vi "Day 8.1 - .vi"(11 "input":i32[][](array[numeric])) -> (3 "output":i16)   [LabVIEW 2021]
panel:
  out "Array":bool[][](array[boolean])
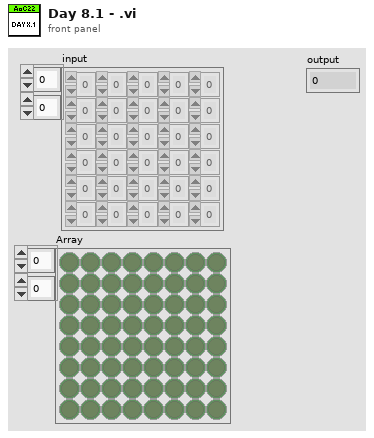
[diagram p1: front panel]
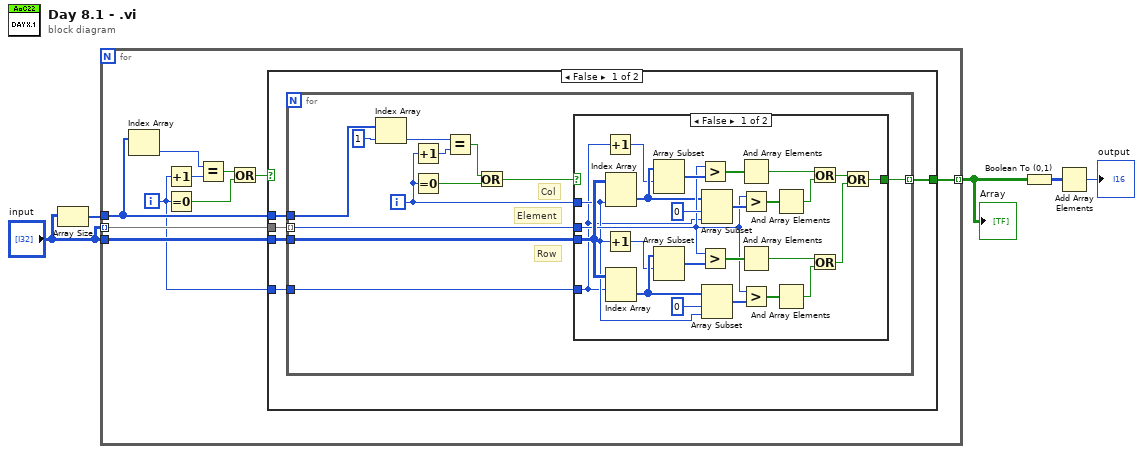
[diagram p0: block diagram]
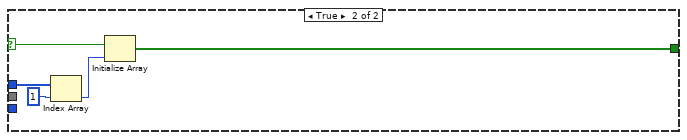
[diagram p3: hidden frame]
diagram:
  n1 = Array Size(array="input") -> (size(s)=w4:i32[])
  n2 = for {
    tunnel: "input" -> [w15] mode=indexing
    tunnel: "input" -> [w14]
    tunnel: w4 -> [w13]
    tunnel: [w7] -> w3 mode=indexing
    i -> [w6]
    n3 = Index Array(array=w13) -> (element=w12:i32)  [unwired: 1 in]
    n4 = Increment(x=w6) -> (x+1=w11:i32)
    n5 = Equal To 0?(x=w6) -> (x = 0?=w9:bool)
    n6 = Equal?(x=w12, y=w11) -> (x = y?=w10:bool)
    n7 = Or(x=w10, y=w9) -> (x .or. y?=w8:bool)
    n8 = case shown="False" w8 {
      selector: w8 -> [_ w63]
      tunnel: w15 -> [w20 _]
      tunnel: w14 -> [w19 _]
      tunnel: w13 -> [w18 w59]
      tunnel: [w17 w62] -> w7
      tunnel: w6 -> [w16 _]
      frame False {
        n9 = for {
          tunnel: w20 -> [w23] mode=indexing
          tunnel: w19 -> [w24]
          tunnel: w18 -> [w28]
          tunnel: [w25] -> w17 mode=indexing
          tunnel: w16 -> [w21]
          i -> [w22]
          # "Col"
          # "Row"
          # "Element"
          n10 = Index Array(array=w28, index=1) -> (element=w29:i32)
          n11 = Increment(x=w22) -> (x+1=w30:i32)
          n12 = Equal To 0?(x=w22) -> (x = 0?=w32:bool)
          n13 = Equal?(x=w29, y=w30) -> (x = y?=w31:bool)
          n14 = Or(x=w31, y=w32) -> (x .or. y?=w26:bool)
          n15 = case shown="False" w26 {
            selector: w26 -> [_ w58]
            tunnel: [w54 w58] -> w25
            tunnel: w24 -> [w57 _]
            tunnel: w23 -> [w47 _]
            tunnel: w22 -> [w34 _]
            tunnel: w21 -> [w33 _]
            frame False {
              n16 = Increment(x=w33) -> (x+1=w36:i32)
              n17 = Increment(x=w34) -> (x+1=w35:i32)
              n18 = Index Array(array=w57, index (col)=w34) -> (element=w38:i32[])  [unwired: 1 in]
              n19 = Index Array(array=w57, index (row)=w33) -> (element=w37:i32[])  [unwired: 1 in]
              n20 = Array Subset(array=w38, index=w36) -> (w51:i32[])  [unwired: 1 in]
              n21 = Array Subset(array=w37, index=w35) -> (w45:i32[])  [unwired: 1 in]
              n22 = Greater?(x=w47, y=w51) -> (0:w56:bool[])
              n23 = Greater?(x=w47, y=w45) -> (0:w55:bool[])
              n24 = Array Subset(array=w38, index=0, length=w33) -> (w50:i32[])
              n25 = Array Subset(array=w37, index=0, length=w34) -> (w44:i32[])
              n26 = And Array Elements(Boolean array=w56) -> (logical AND=w40:bool)
              n27 = Greater?(x=w47, y=w50) -> (0:w52:bool[])
              n28 = And Array Elements(Boolean array=w55) -> (logical AND=w43:bool)
              n29 = Greater?(x=w47, y=w44) -> (0:w48:bool[])
              n30 = And Array Elements(Boolean array=w52) -> (logical AND=w49:bool)
              n31 = And Array Elements(Boolean array=w48) -> (logical AND=w42:bool)
              n32 = Or(x=w40, y=w49) -> (x .or. y?=w39:bool)
              n33 = Or(x=w43, y=w42) -> (x .or. y?=w41:bool)
              n34 = Or(x=w39, y=w41) -> (x .or. y?=w54:bool)
            }
            frame True {
            }
          }
        }
      }
      frame True {
        n35 = Index Array(array=w59, index=1) -> (element=w60:i32)
        n36 = Initialize Array(w63, w60) -> (w62:bool[])
      }
    }
  }
  "Array" <- w3
  n37 = Boolean To (0,1)(Boolean=w3) -> (0, 1=w2:i16[][])
  n38 = Add Array Elements(numeric array=w2) -> (sum=→"output":i16)
